vi "TagDB Refmgr-Load Rule csv.vi"(8 "error in (no error)":errorcluster, 11 "Path":path) -> (0 "error out":errorcluster, 3 "Array 2":T1[](array[typedef]))   [LabVIEW 2017, in "UIStateExpression.lvlib"]
uses:
  UIStateExpression/UIStateExpression.lvlib
  Typedef/RefMgr-Logic-State.ctl
  Typedef/RefMgr-StateChangeType.ctl
  <userlib>/NEVSTOP-Programming-Palette/Configuration/ClusterCfgTable/ClusterCfgTable_nevstop.lvlib
  TagDB RefManager.lvlib
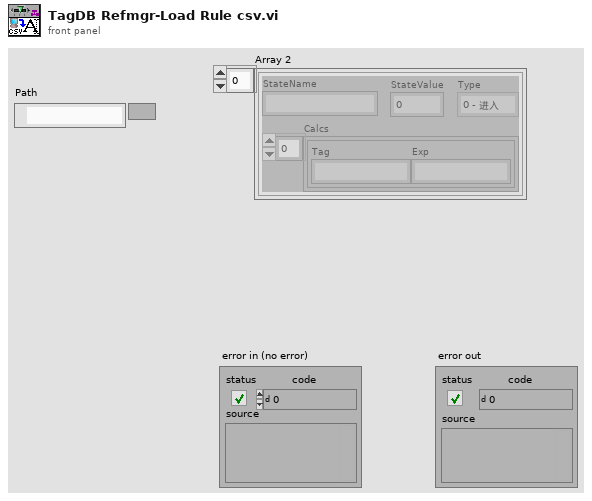
[diagram p1: front panel]
types:
  T1 = typedef "TagDB RefManager.lvlib/RefMgr-Logic-State.ctl" = cluster{"StateName":string, "StateValue":i32, "Type":T2, "Calcs":cluster{"Tag":string, "Exp":string}[]}
  T2 = typedef "TagDB RefManager.lvlib/RefMgr-StateChangeType.ctl" = enum16{"0 - 进入", "1 - 等于", "2 - 退出"}
  T3 = enum16{"open", "replace", "create", "open or create", "replace or create", "replace or create with confirmation"}
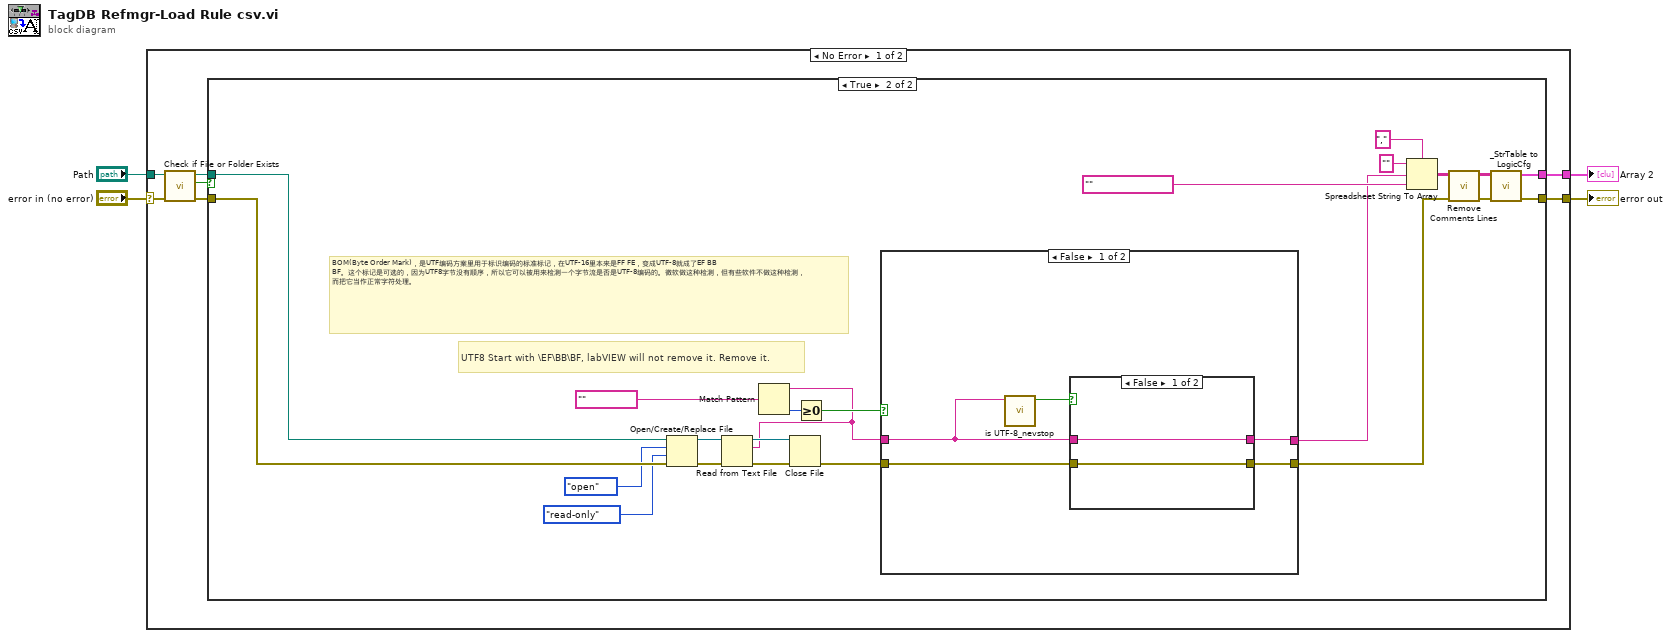
[diagram p0: block diagram]
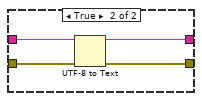
[diagram p3: hidden frame]
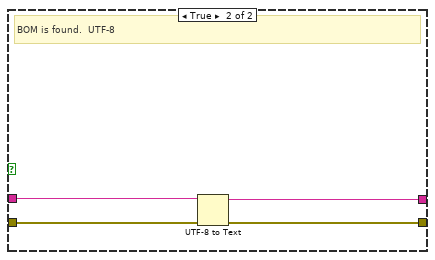
[diagram p4: hidden frame]
diagram:
  n1 = case shown="No Error" "error in (no error)" {
    selector: "error in (no error)" -> [w9 w51]
    tunnel: "Path" -> [w11 _]
    tunnel: [w7 w51] -> w2
    tunnel: [w6 _] -> w1
    frame No Error {
      n2 = call <vilib>:"Check if File or Folder Exists.vi"("error in (no error)"=w9, "path"=w11) -> ("error out"=w8:errorcluster, "file or folder exists?"=w5:bool, "dup path"=w10:path)  [unwired: 7 in]
      n3 = case shown="True" w5 {
        tunnel: w10 -> [_ w35]
        tunnel: w8 -> [w12 w34]
        tunnel: [w12 w31] -> w7
        tunnel: [_ w30] -> w6
        frame False {
        }
        frame True {
          # "BOM(Byte Order Mark)，是UTF编码方案里用于标识编码的标准标记，在UTF-16里本来是FF FE，变成UTF-8就成了EF BB BF。这个标记是可选的，因为UTF8字节没有顺序，所以它可以被用来检测一个字节流是否是UTF-8编码的。微软做这种检测，但有些软件不做这种检测， 而把它当作正常字符处理。"
          # "UTF8 Start with \\EF\\BB\\BF, labVIEW will not remove it. Remove it."
          n4 = Open/Create/Replace File(file path (use dialog)=w35, error in=w34, operation (0:open)=T3."open", access (0:read/write)=enum16{"read/write", "read-only", "write-only"}."read-only") -> (refnum out=w21:refnum<file>, error out=w18:errorcluster)  [unwired: 2 in, 1 out]
          n5 = Read from Text File(file (use dialog)=w21, error in=w18) -> (refnum out=w20:refnum<file>, text=w13:string, error out=w19:errorcluster)  [unwired: 2 in, 1 out]
          n6 = Match Pattern(string=w13, regular expression="﻿") -> (offset past match=w17:i32)  [unwired: 1 in, 3 out]
          n7 = Close File(refnum=w20, error in=w19) -> (error out=w14:errorcluster)  [unwired: 1 out]
          n8 = Greater Or Equal To 0?(x=w17) -> (x >= 0?=w16:bool)
          n9 = case shown="False" w16 {
            tunnel: [w39 w49] -> w32
            tunnel: w13 -> [w38 w50]
            tunnel: w14 -> [w36 w48]
            tunnel: [w37 w47] -> w24
            frame False {
              n10 = call <userlib>:"is UTF-8_nevstop.vi"("String"=w38) -> ("UTF8"=w40:bool)  [unwired: 10 in]
              n11 = case shown="False" w40 {
                tunnel: w38 -> [w41 w46]
                tunnel: [w41 w45] -> w39
                tunnel: w36 -> [w42 w44]
                tunnel: [w42 w43] -> w37
                frame False {
                }
                frame True {
                  n12 = UTF-8 to Text(8:w44, 11:w46) -> (0:w43:errorcluster, 3:w45:string)  [unwired: 1 in]
                }
              }
            }
            frame True {
              # "BOM is found.  UTF-8"
              n13 = UTF-8 to Text(8:w48, 11:w50) -> (0:w47:errorcluster, 3:w49:string)  [unwired: 1 in]
            }
          }
          n14 = Spreadsheet String To Array(delimiter (Tab)=",", format string="", spreadsheet string=w32, array type (2D Dbl)="" ("spreadsheet string")) -> (array=w27:string[][])
          n15 = call <userlib>:"Remove Comments Lines.vi"("error in (no error)"=w24, "CfgTable in"=w27) -> ("error out"=w25:errorcluster, "CfgTable out"=w26:string[][])  [unwired: 8 in]
          n16 = call "_StrTable to LogicCfg.vi"("error in (no error)"=w25, "CfgTable in"=w26) -> ("error out"=w31:errorcluster, "Array 2"=w30:T1[])  [unwired: 8 in]
        }
      }
    }
    frame Error {
    }
  }
  "error out" <- w2
  "Array 2" <- w1
